vi "Launch Dialog.vi"(4 "Dialog Type":refnum<class "ITest Executive Builder Dialog.lvclass">, 6 "Unique ID":string, 8 "error in (no error)":errorcluster, 11 "Test Executive Builder in":refnum<class "Test Executive Builder.lvclass">) -> (0 "error out":errorcluster, 3 "Test Executive Builder out":refnum<class "Test Executive Builder.lvclass">)   [LabVIEW 2019, in "Test Executive Builder.lvclass"]
uses:
  <vilib>/gpm_packages/@cs/Test-executive-builder/Example/Application/Test Executive Builder/Test Executive Builder/Test Executive Builder.lvclass
  C:/Program Files/National Instruments/LabVIEW 2019/vi.lib/gpm_packages/@cs/Test-executive-builder/Source/Test Executive Builder Model/Test Executive Builder Model/Test Executive Builder Model.lvclass
  C:/Program Files/National Instruments/LabVIEW 2019/vi.lib/ActorFramework/Actor/Actor.lvclass
  C:/Program Files/National Instruments/LabVIEW 2019/vi.lib/gpm_packages/@cs/mva-core/Source/IObserver/IObserver/IObserver.lvclass
  <vilib>/gpm_packages/@cs/Test-executive-builder/Source/Test Executive Builder Dialogs/ITest Executive Builder Dialog/ITest Executive Builder Dialog.lvclass
  <vilib>/gpm_packages/@cs/Test-executive-builder/Example/Application/Test Executive Builder/Test Executive Builder/Test Executive Builder.lvclass/Test Executive Builder.ctl
  <vilib>/gpm_packages/@cs/Test-executive-builder/Source/Test Executive Builder Model/Test Executive Builder Model/Test Executive Builder Model.lvclass/Test Executive Builder Model.ctl
  <vilib>/gpm_packages/@cs/Test-executive-builder/Source/Test Executive Builder Dialogs/ITest Executive Builder Dialog/ITest Executive Builder Dialog.lvclass/ITest Executive Builder Dialog.ctl
  <vilib>/ActorFramework/Message Enqueuer/Message Enqueuer.lvclass/Message Enqueuer.ctl
  <vilib>/gpm_packages/@cs/mva-core/Source/IObserver/IObserver/IObserver.lvclass/IObserver.ctl
  <vilib>/ActorFramework/Message Enqueuer/Enqueue.vi
  <vilib>/ActorFramework/Stop Msg/Stop Msg.lvclass
  C:/Program Files/National Instruments/LabVIEW 2019/vi.lib/ActorFramework/Message/Message.lvclass
  <vilib>/ActorFramework/Message Priority Queue/Priority Enqueue.vi
  <vilib>/gpm_packages/@cs/Test-executive-builder/Source/Test Executive Builder Model/Test Executive Builder Model/Test Executive Builder Model.lvclass
  <vilib>/ActorFramework/Actor/Actor.lvclass
  <vilib>/gpm_packages/@cs/mva-core/Source/IObserver/IObserver/IObserver.lvclass
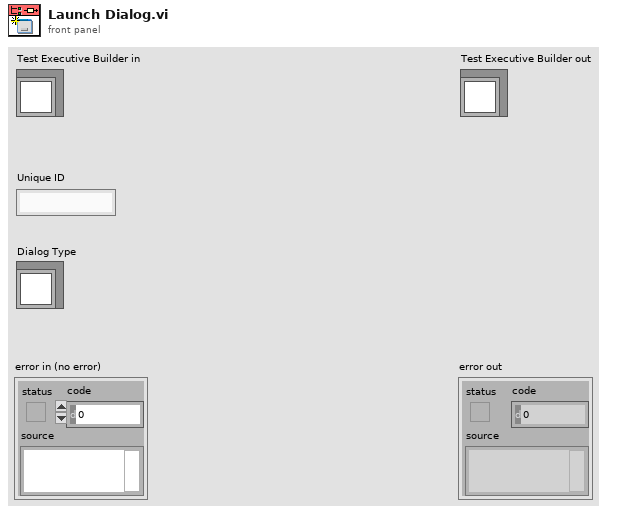
[diagram p1: front panel]
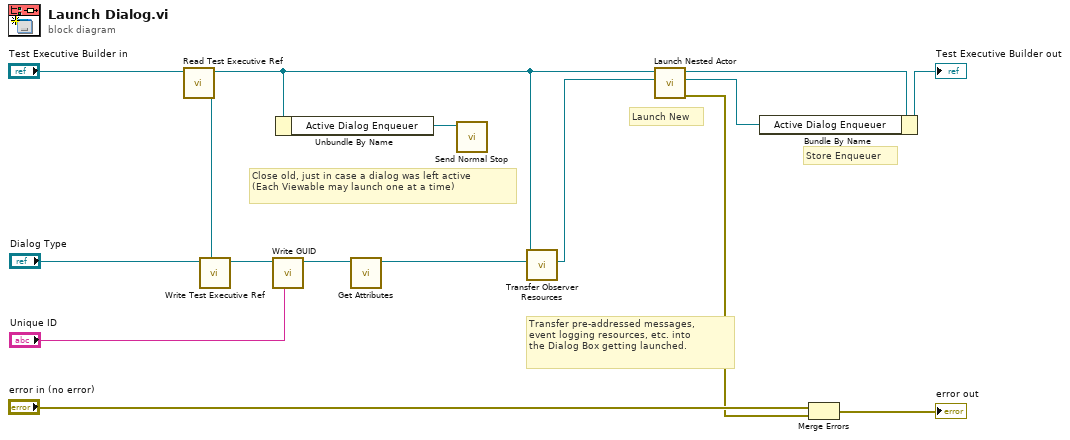
[diagram p0: block diagram]
diagram:
  # "Store Enqueuer"
  # "Launch New"
  # "Close old, just in case a dialog was left active\n(Each Viewable may launch one at a time)"
  # "Transfer pre-addressed messages,\nevent logging resources, etc. into\nthe Dialog Box getting launched."
  n1 = call <vilib>:"Read Test Executive Ref.vi"("Test Executive Builder Model in"="Test Executive Builder in") -> ("Test Executive Ref"=w13:refnum<data-value>, "Test Executive Builder Model out"=w8:refnum<class "Test Executive Builder.lvclass">)  [unwired: 9 in]
  n2 = call <vilib>:"Write Test Executive Ref.vi"("Test Executive Ref"=w13, "ITest Executive Builder Dialog in"="Dialog Type") -> ("ITest Executive Builder Dialog out"=w12:refnum<class "ITest Executive Builder Dialog.lvclass">)  [unwired: 9 in]
  n3 = call <vilib>:"Write GUID.vi"("GUID"="Unique ID", "ITest Executive Builder Dialog in"=w12) -> ("ITest Executive Builder Dialog out"=w10:refnum<class "ITest Executive Builder Dialog.lvclass">)  [unwired: 9 in]
  n4 = Unbundle By Name(w8) -> ("Active Dialog Enqueuer"=w9:refnum<class "Message Enqueuer.lvclass">)
  n5 = call-dynamic "Get Attributes.vi"("ITest Executive Builder Dialog in"=w10) -> ("ITest Executive Builder Dialog out"=w7:refnum<class "ITest Executive Builder Dialog.lvclass">)  [unwired: 9 in, 1 out]
  n6 = call <vilib>:"Send Normal Stop.vi"("Message Enqueuer"=w9) -> ()  [unwired: 10 in, 1 out]
  n7 = call <vilib>:"Transfer Observer Resources.vi"("Recipient Observer In"=w7, "Running Observer"=w8) -> ("Recipient Observer Out"=w6:refnum<class "ITest Executive Builder Dialog.lvclass">)  [unwired: 9 in]
  n8 = call <vilib>:"Launch Nested Actor.vi"("Nested Actor"=w6, "Caller Actor in"=w8) -> ("error out"=w1:errorcluster, "Nested Actor's Enqueuer"=w3:refnum<class "Message Enqueuer.lvclass">, "Caller Actor out"=w5:refnum<class "Test Executive Builder.lvclass">)  [unwired: 7 in]
  n9 = Bundle By Name(cluster=w5, "Active Dialog Enqueuer"=w3) -> (→"Test Executive Builder out":refnum<class "Test Executive Builder.lvclass">)
  n10 = Merge Errors("error in (no error)", w1) -> (→"error out":errorcluster)
